vi "Read_Lock.vi"() -> ()   [LabVIEW 2019]
uses:
  Components/MeasurementConfigGlobals.vi
  Components/ReadLockGlobals.vi
panel:
  out "VISA":refnum<visa-resource-name>
  out "VISA":refnum<visa-resource-name>
  out "Phase":dbl
  in  "Sens2":T1(ring)
  out "Sens Read 2":dbl
  out "V 2":dbl
  out "Phase":dbl
  in  "Sens":T1(ring)
  out "Sens Read":dbl
  out "V":dbl
  # "Lockin- 1"
  # "Lockin- 2"
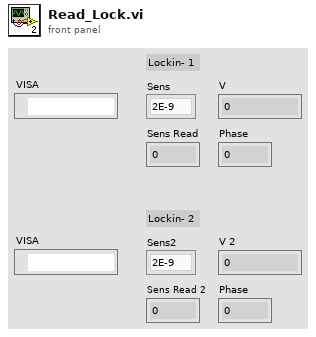
[diagram p1: front panel]
types:
  T1 = enum16{"2E-9", "5E-9", "1E-8", "2E-8", "5E-8", "1E-7", "2E-7", "5E-7", "1E-6", "2E-6", "5E-6", "1E-5", "2E-5", "5E-5", "1E-4", "2E-4", "5E-4", "1E-3", "2E-3", "5E-3", "1E-2", "2E-2", "5E-2", "1E-1", "2E-1", "5E-1", "1"}
  T2 = cluster{"Name":string, "Measurment Type":string, "I Max":dbl, "Freq/Delay":dbl, "Address":refnum<visa-resource-name>, "Enabled":bool}[]
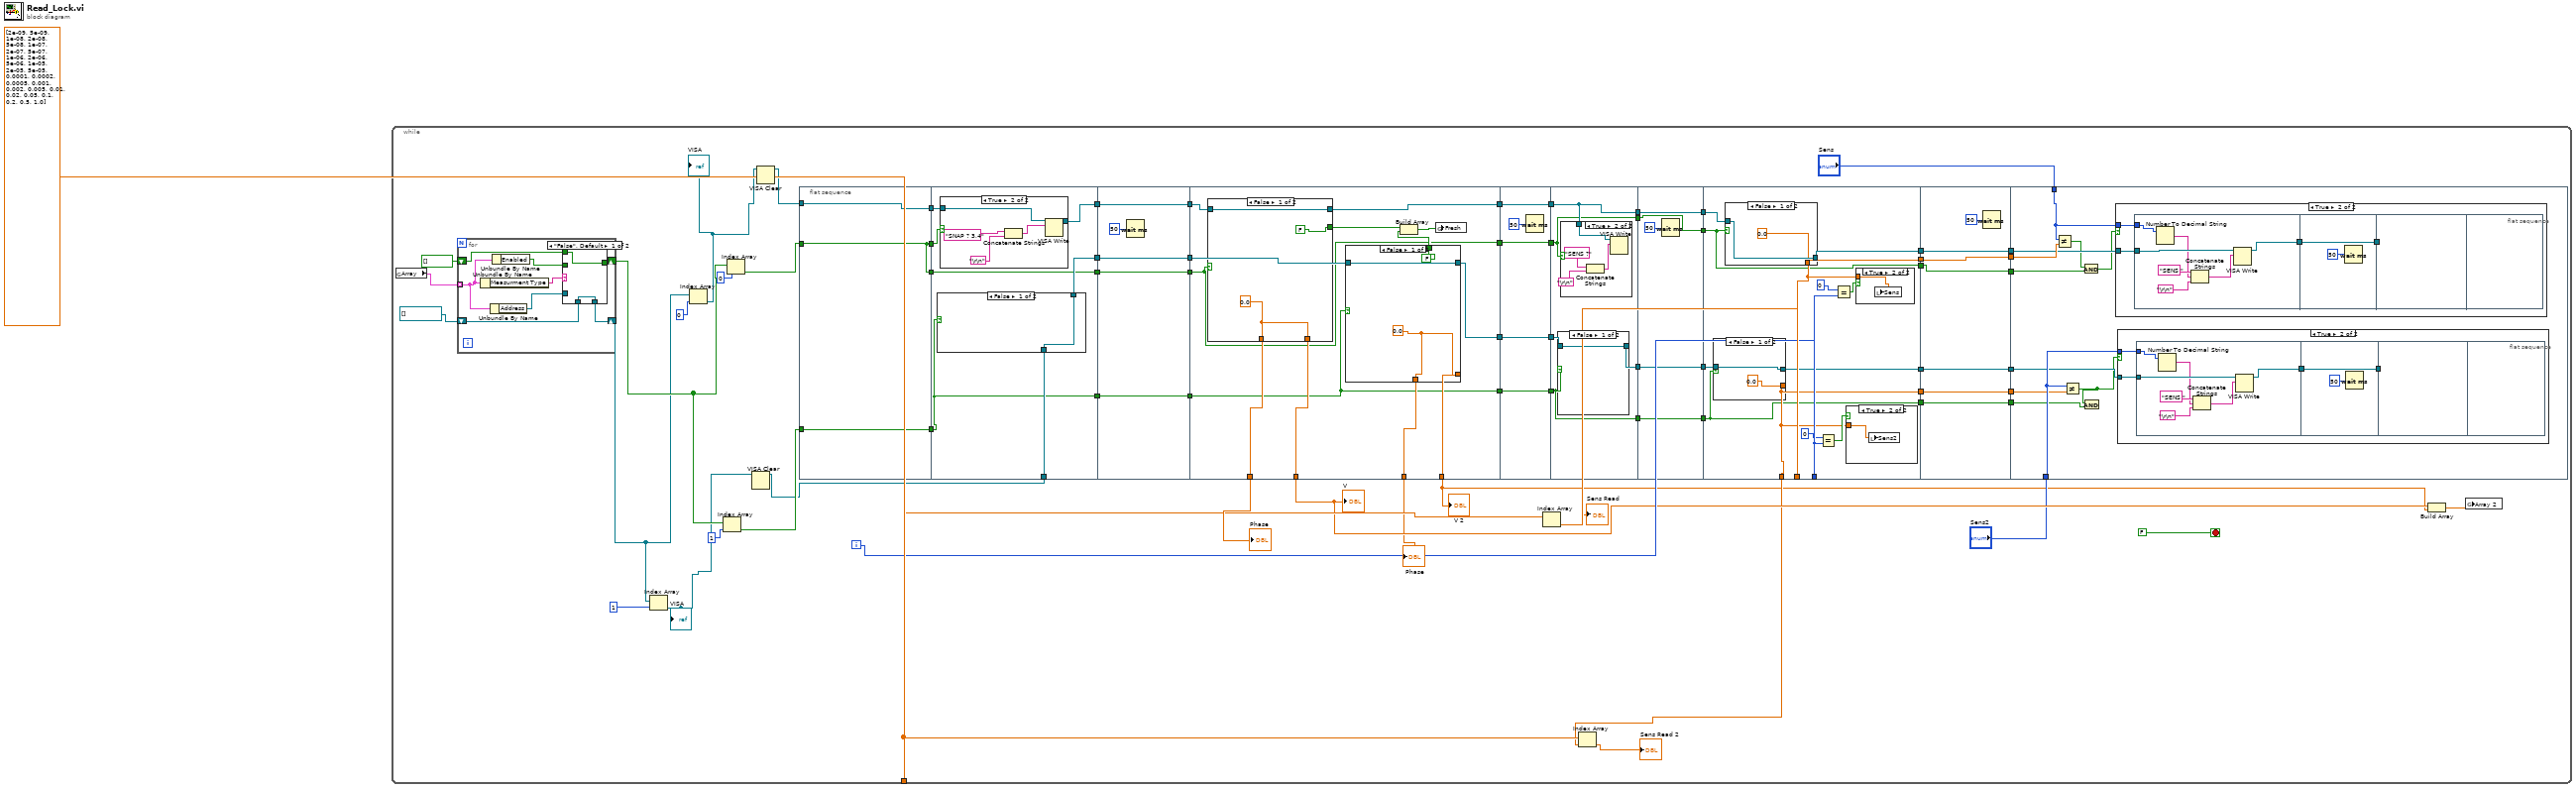
[diagram p0: block diagram]
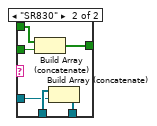
[diagram p2: hidden frame]
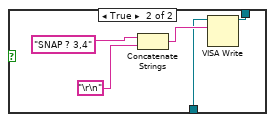
[diagram p3: hidden frame]
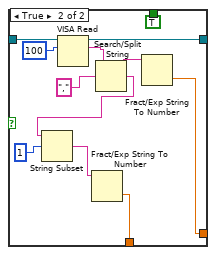
[diagram p5: hidden frame]
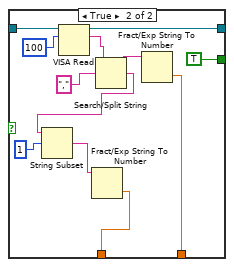
[diagram p6: hidden frame]
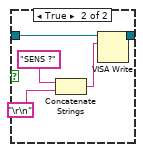
[diagram p7: hidden frame]
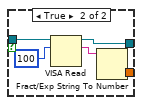
[diagram p9: hidden frame]
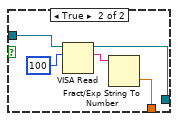
[diagram p10: hidden frame]
diagram:
  n1 = while {
    tunnel: dbl[] [2e-09, 5e-09, 1e-08, 2e-08, 5e-08, 1e-07, 2e-07, 5e-07, 1e-06, 2e-06, 5e-06, 1e-05, 2e-05, 5e-05, 0.0001, 0.0002, 0.0005, 0.001, 0.002, 0.005, 0.01, 0.02, 0.05, 0.1, 0.2, 0.5, 1.0] -> [w53]
    i -> [w54]
    stop <- FALSE stop-if-true
    n2 = global read "MeasurementConfigGlobals.vi" "Array"() -> (w14:T2)
    n3 = for {
      tunnel: w14 -> [w74] mode=indexing
      shift-right: [w75] -> w15
      shift-left: refnum<visa-resource-name>[] [] -> [w77]
      shift-right: [w71] -> w16
      shift-left: bool[] [] -> [w73]
      n4 = Unbundle By Name(w74) -> ("Measurment Type"=w78:string)
      n5 = Unbundle By Name(w74) -> ("Address"=w76:refnum<visa-resource-name>)
      n6 = Unbundle By Name(w74) -> ("Enabled"=w72:bool)
      n7 = case shown="\"False\", Default" w78 {
        tunnel: w77 -> [w80 w86]
        tunnel: w76 -> [_ w85]
        tunnel: [w80 w84] -> w75
        tunnel: w73 -> [w79 w83]
        tunnel: w72 -> [_ w82]
        tunnel: [w79 w81] -> w71
        frame "False", Default {
        }
        frame "SR830" {
          n8 = Build Array (concatenate)(w83, w82) -> (w81:bool[])
          n9 = Build Array (concatenate)(w86, w85) -> (w84:refnum<visa-resource-name>[])
        }
      }
    }
    n10 = Index Array(array=w15, index=1) -> (element=w2:refnum<visa-resource-name>)
    "VISA" <- w2
    n11 = Index Array(array=w15, index=0) -> (element=w5:refnum<visa-resource-name>)
    "VISA" <- w5
    n12 = Index Array(array=w16, index=1) -> (element=w8:bool)
    n13 = Index Array(array=w16, index=0) -> (element=w7:bool)
    n14 = VISA Clear(VISA resource name=w2) -> (VISA resource name out=w3:refnum<visa-resource-name>)  [unwired: 1 in, 1 out]
    n15 = VISA Clear(VISA resource name=w5) -> (VISA resource name out=w4:refnum<visa-resource-name>)  [unwired: 1 in, 1 out]
    n16 = flat-sequence {
      tunnel: [w89] -> w55
      tunnel: w4 -> [w89]
      tunnel: [w87] -> w35
      tunnel: w7 -> [w87]
      tunnel: [w88] -> w34
      tunnel: w8 -> [w88]
      tunnel: [w87] -> w33
      tunnel: [w96] -> w70
      tunnel: w55 -> [w95]
      tunnel: w3 -> [w94]
      tunnel: [w93] -> w48
      tunnel: w35 -> [w92]
      tunnel: w34 -> [w90]
      tunnel: w33 -> [w91]
      tunnel: [w91] -> w32
      tunnel: [w90] -> w29
      tunnel: w70 -> [w113]
      tunnel: [w113] -> w69
      tunnel: w48 -> [w111]
      tunnel: [w111] -> w47
      tunnel: w32 -> [w110]
      tunnel: [w110] -> w31
      tunnel: [w109] -> w30
      tunnel: w29 -> [w109]
      tunnel: w69 -> [w126]
      tunnel: [w125] -> w68
      tunnel: [w124] -> w51
      tunnel: [w123] -> w56
      tunnel: [w122] -> w49
      tunnel: [w121] -> w36
      tunnel: w47 -> [w120]
      tunnel: [w118] -> w46
      tunnel: w31 -> [w115]
      tunnel: w30 -> [w114]
      tunnel: [w115] -> w28
      tunnel: [w114] -> w25
      tunnel: w68 -> [w160]
      tunnel: [w160] -> w67
      tunnel: w46 -> [w159]
      tunnel: [w159] -> w45
      tunnel: w28 -> [w158]
      tunnel: [w158] -> w27
      tunnel: [w157] -> w26
      tunnel: w25 -> [w157]
      tunnel: w67 -> [w166]
      tunnel: [w166] -> w66
      tunnel: w45 -> [w165]
      tunnel: [w164] -> w43
      tunnel: w27 -> [w162]
      tunnel: w26 -> [w163]
      tunnel: [w163] -> w22
      tunnel: [w162] -> w19
      tunnel: w66 -> [w180]
      tunnel: [w180] -> w65
      tunnel: [w179] -> w44
      tunnel: w43 -> [w179]
      tunnel: w22 -> [w178]
      tunnel: [w178] -> w21
      tunnel: [w177] -> w20
      tunnel: w19 -> [w177]
      tunnel: w65 -> [w194]
      tunnel: [w190] -> w63
      tunnel: [w190] -> w61
      tunnel: [w193] -> w59
      tunnel: w54 -> [w187]
      tunnel: w44 -> [w188]
      tunnel: [w185] -> w42
      tunnel: [w185] -> w40
      tunnel: [w184] -> w37
      tunnel: [w183] -> w24
      tunnel: w21 -> [w183]
      tunnel: w20 -> [w182]
      tunnel: [w182] -> w17
      tunnel: [w216] -> w62
      tunnel: w61 -> [w216]
      tunnel: [w215] -> w60
      tunnel: w59 -> [w215]
      tunnel: w40 -> [w214]
      tunnel: [w214] -> w39
      tunnel: [w213] -> w38
      tunnel: w37 -> [w213]
      tunnel: w24 -> [w212]
      tunnel: [w212] -> w23
      tunnel: [w211] -> w18
      tunnel: w17 -> [w211]
      tunnel: w62 -> [w228]
      tunnel: w60 -> [w227]
      tunnel: "Sens" -> [w226]
      tunnel: "Sens2" -> [w225]
      tunnel: w39 -> [w224]
      tunnel: w38 -> [w223]
      tunnel: w23 -> [w221]
      tunnel: w18 -> [w218]
      frame #0 {
      }
      frame #1 {
        n17 = case shown="False" w90 {
          tunnel: w94 -> [w97 w99]
          tunnel: [w97 w98] -> w93
          frame False {
          }
          frame True {
            n18 = Concatenate Strings("SNAP ? 3,4", "\r\n") -> (w101:string)
            n19 = VISA Write(VISA resource name=w99, write buffer=w101) -> (VISA resource name out=w98:refnum<visa-resource-name>)  [unwired: 1 in, 2 out]
          }
        }
        n20 = case shown="True" w92 {
          tunnel: [w103 w108] -> w96
          tunnel: w95 -> [w103 w105]
          frame False {
          }
          frame True {
            n21 = Concatenate Strings("SNAP ? 3,4", "\r\n") -> (w106:string)
            n22 = VISA Write(VISA resource name=w105, write buffer=w106) -> (VISA resource name out=w108:refnum<visa-resource-name>)  [unwired: 1 in, 2 out]
          }
        }
      }
      frame #2 {
        n23 = Wait (ms)(milliseconds to wait=50) -> ()  [unwired: 1 out]
      }
      frame #3 {
        n24 = case shown="False" w115 {
          tunnel: w126 -> [w144 w152]
          tunnel: [w144 w151] -> w125
          tunnel: [w143 w150] -> w124
          tunnel: [w143 w146] -> w123
          tunnel: [FALSE TRUE] -> w117
          frame False {
            w143 = 0.0
          }
          frame True {
            n25 = VISA Read(VISA resource name=w152, byte count=u32 100) -> (VISA resource name out=w151:refnum<visa-resource-name>, read buffer=w153:string)  [unwired: 1 in, 2 out]
            n26 = Search/Split String(string=w153, search string/char (-)=",") -> (substring before match=w155:string, match + rest of string=w149:string)  [unwired: 1 in, 1 out]
            n27 = String Subset(string=w149, offset (0)=1) -> (substring=w147:string)  [unwired: 1 in]
            n28 = Fract/Exp String To Number(string=w147) -> (number=w146:dbl)  [unwired: 1 in, 3 out]
            n29 = Fract/Exp String To Number(string=w155) -> (number=w150:dbl)  [unwired: 1 in, 3 out]
          }
        }
        n30 = case shown="False" w114 {
          tunnel: [w128 w134] -> w122
          tunnel: [w128 w133] -> w121
          tunnel: w120 -> [w129 w132]
          tunnel: [w129 w131] -> w118
          tunnel: [FALSE TRUE] -> w116
          frame False {
            w128 = 0.0
          }
          frame True {
            n31 = VISA Read(VISA resource name=w132, byte count=u32 100) -> (VISA resource name out=w131:refnum<visa-resource-name>, read buffer=w138:string)  [unwired: 1 in, 2 out]
            n32 = Search/Split String(string=w138, search string/char (-)=",") -> (substring before match=w140:string, match + rest of string=w137:string)  [unwired: 1 in, 1 out]
            n33 = String Subset(string=w137, offset (0)=1) -> (substring=w135:string)  [unwired: 1 in]
            n34 = Fract/Exp String To Number(string=w135) -> (number=w134:dbl)  [unwired: 1 in, 3 out]
            n35 = Fract/Exp String To Number(string=w140) -> (number=w133:dbl)  [unwired: 1 in, 3 out]
          }
        }
        n36 = Build Array(w117, w116) -> (w119:bool[])
        n37 = global write "ReadLockGlobals.vi" "Fresh"(w119) -> ()
      }
      frame #4 {
        n38 = Wait (ms)(milliseconds to wait=50) -> ()  [unwired: 1 out]
      }
      frame #5 {
        n39 = case shown="False" w163 {
          tunnel: w165 -> [w167 w169]
          tunnel: [w167 w168] -> w164
          frame False {
          }
          frame True {
            n40 = Concatenate Strings("SENS ?", "\r\n") -> (w171:string)
            n41 = VISA Write(VISA resource name=w169, write buffer=w171) -> (VISA resource name out=w168:refnum<visa-resource-name>)  [unwired: 1 in, 2 out]
          }
        }
        n42 = case shown="True" w162 {
          tunnel: w166 -> [_ w174]
          frame False {
          }
          frame True {
            n43 = Concatenate Strings("SENS ?", "\r\n") -> (w175:string)
            n44 = VISA Write(VISA resource name=w174, write buffer=w175) -> ()  [unwired: 1 in, 3 out]
          }
        }
      }
      frame #6 {
        n45 = Wait (ms)(milliseconds to wait=50) -> ()  [unwired: 1 out]
      }
      frame #7 {
        n46 = case shown="False" w183 {
          tunnel: w188 -> [w196 w199]
          tunnel: [0.0 w198] -> w185
          tunnel: [w196 w197] -> w184
          frame False {
          }
          frame True {
            n47 = VISA Read(VISA resource name=w199, byte count=u32 100) -> (VISA resource name out=w197:refnum<visa-resource-name>, read buffer=w200:string)  [unwired: 1 in, 2 out]
            n48 = Fract/Exp String To Number(string=w200) -> (number=w198:dbl)  [unwired: 1 in, 3 out]
          }
        }
        n49 = case shown="False" w182 {
          tunnel: w194 -> [w203 w208]
          tunnel: [w203 w205] -> w193
          tunnel: [0.0 w204] -> w190
          frame False {
          }
          frame True {
            n50 = VISA Read(VISA resource name=w208, byte count=u32 100) -> (VISA resource name out=w205:refnum<visa-resource-name>, read buffer=w206:string)  [unwired: 1 in, 2 out]
            n51 = Fract/Exp String To Number(string=w206) -> (number=w204:dbl)  [unwired: 1 in, 3 out]
          }
        }
        n52 = Equal?(x=0, y=w187) -> (x = y?=w186:bool)
        n53 = Equal?(x=0, y=w187) -> (x = y?=w191:bool)
        n54 = case shown="True" w186 {
          tunnel: w185 -> [_ w209]
          frame False {
          }
          frame True {
            n55 = local write "Sens2"(w209) -> ()
          }
        }
        n56 = case shown="True" w191 {
          tunnel: w190 -> [_ w210]
          frame False {
          }
          frame True {
            n57 = local write "Sens"(w210) -> ()
          }
        }
      }
      frame #8 {
        n58 = Wait (ms)(milliseconds to wait=50) -> ()  [unwired: 1 out]
      }
      frame #9 {
        n59 = Not Equal?(x=w226, y=w228) -> (x != y?=w219:bool)
        n60 = Not Equal?(x=w225, y=w224) -> (x != y?=w222:bool)
        n61 = And(x=w219, y=w218) -> (x .and. y?=w220:bool)
        n62 = And(x=w222, y=w221) -> ()  [unwired: 1 out]
        n63 = case shown="True" w220 {
          tunnel: w227 -> [_ w245]
          tunnel: w226 -> [_ w244]
          frame False {
          }
          frame True {
            n64 = flat-sequence {
              tunnel: w245 -> [w252]
              tunnel: w244 -> [w250]
              tunnel: [w247] -> w242
              tunnel: [w253] -> w243
              tunnel: w242 -> [w253]
              tunnel: w243 -> [_]
              frame #0 {
                n65 = Number To Decimal String(number=w250) -> (decimal integer string=w249:string)  [unwired: 1 in]
                n66 = Concatenate Strings("SENS ", w249, "\r\n") -> (w248:string)
                n67 = VISA Write(VISA resource name=w252, write buffer=w248) -> (VISA resource name out=w247:refnum<visa-resource-name>)  [unwired: 1 in, 2 out]
              }
              frame #1 {
                n68 = Wait (ms)(milliseconds to wait=50) -> ()  [unwired: 1 out]
              }
              frame #2 {
              }
              frame #3 {
              }
            }
          }
        }
        n69 = case shown="True" w222 {
          tunnel: w223 -> [_ w232]
          tunnel: w225 -> [_ w231]
          frame False {
          }
          frame True {
            n70 = flat-sequence {
              tunnel: w232 -> [w239]
              tunnel: w231 -> [w237]
              tunnel: [w234] -> w229
              tunnel: [w240] -> w230
              tunnel: w229 -> [w240]
              tunnel: w230 -> [_]
              frame #0 {
                n71 = Number To Decimal String(number=w237) -> (decimal integer string=w236:string)  [unwired: 1 in]
                n72 = Concatenate Strings("SENS ", w236, "\r\n") -> (w235:string)
                n73 = VISA Write(VISA resource name=w239, write buffer=w235) -> (VISA resource name out=w234:refnum<visa-resource-name>)  [unwired: 1 in, 2 out]
              }
              frame #1 {
                n74 = Wait (ms)(milliseconds to wait=50) -> ()  [unwired: 1 out]
              }
              frame #2 {
              }
              frame #3 {
              }
            }
          }
        }
      }
    }
    n75 = Index Array(array=w53, index=w63) -> (element=→"Sens Read":dbl)
    n76 = Index Array(array=w53, index=w42) -> (element=→"Sens Read 2":dbl)
    n77 = Build Array(w51, w36) -> (w50:dbl[])
    n78 = global write "ReadLockGlobals.vi" "Array 2"(w50) -> ()
    "V" <- w51
    "Phase" <- w56
    "V 2" <- w36
    "Phase" <- w49
  }
